vi "writeToSerialPort.vi"(1 "Cmmd":string="*idn?", 2 "input COM Port":refnum<visa-resource-name>="COM10") -> (0 "data written to port?":bool=TRUE)   [LabVIEW 2015]
panel:
  out "read buffer":string="\n"
  in  "milliseconds to wait":u32=1000
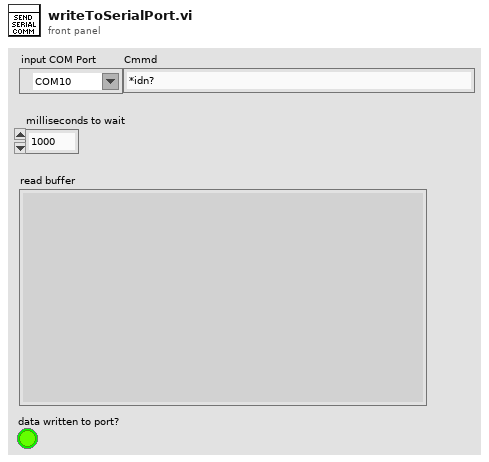
[diagram p1: front panel]
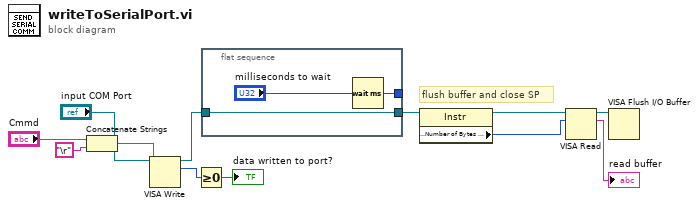
[diagram p0: block diagram]
diagram:
  # "flush buffer and close SP"
  n1 = Concatenate Strings("Cmmd", "\r") -> (w1:string)
  n2 = VISA Write(VISA resource name="input COM Port", write buffer=w1) -> (VISA resource name out=w3:refnum<visa-resource-name>, return count=w5:u32)  [unwired: 1 in, 1 out]
  n3 = Greater Or Equal To 0?(x=w5) -> (x >= 0?=→"data written to port?":bool)
  n4 = flat-sequence {
    tunnel: w3 -> [w15]
    tunnel: [w15] -> w10
    tunnel: [w13] -> _
    frame #0 {
      n5 = Wait (ms)(milliseconds to wait="milliseconds to wait") -> (millisecond timer value=w13:u32)
    }
  }
  n6 = property class="Instr"(reference=w10) -> (reference out=w11:refnum<visa-resource-name>, "Serial Settings:Number of Bytes at Serial Port"=w9:u32)  [unwired: 1 in, 1 out]
  n7 = VISA Read(VISA resource name=w11, byte count=w9) -> (VISA resource name out=w12:refnum<visa-resource-name>, read buffer=→"read buffer":string)  [unwired: 1 in, 2 out]
  n8 = VISA Flush I/O Buffer(VISA resource name=w12) -> ()  [unwired: 2 in, 2 out]
